vi "Ends With.vi"() -> ()   [LabVIEW 2017, in "Transparent Assertions.Tests.lvlib" / "Assert String Ends With.lvlib"]
uses:
  Assert String Ends With.lvlib
  src/Transparent Assertions/Transparent Assertions.lvlib
panel:
  out "error out":errorcluster
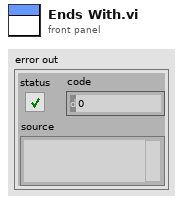
[diagram p1: front panel]
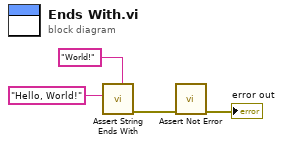
[diagram p0: block diagram]
diagram:
  n1 = call "Assert String Ends With.vi"("Suffix"="World!", "String"="Hello, World!") -> ("error out"=w2:errorcluster)  [unwired: 9 in]
  n2 = call "Assert Not Error.vi"("error in (no error)"=w2) -> ("error out"=→"error out":errorcluster)  [unwired: 10 in]
